vi "ACT_CLOSE.vi"(7 "StateValveModbus":T1=enum."CLOSING", 8 "error in (no error)":errorcluster, 11 "NeedleValve in":refnum<class "NeedleValve.lvclass">) -> (0 "error out":errorcluster, 3 "NeedleValve out":refnum<class "NeedleValve.lvclass">)   [LabVIEW 2019, in "NeedleValve.lvclass"]
uses:
  NeedleValve.lvclass
  TypeDef/Needle Valve State.ctl
  NeedleValve.lvclass/NeedleValve.ctl
  modbus engine custom/MB_ENGINE_class/cmd enum.ctl
  ef2003b6-d044-46f0-abe2-5d2387dde1d8.vi
  432cf372-d557-43cf-ab82-687c716dd17b.vi
  9ce69719-d540-4c82-92ba-c0e5243c761a.vi
  78836dd0-8225-4459-8d70-d600215e9411.vi
  modbus engine custom/MB_ENGINE_class/MB_ENGINE.lvclass
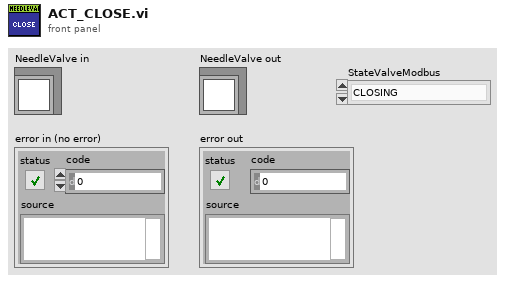
[diagram p1: front panel]
types:
  T1 = typedef "Needle Valve State.ctl" = enum16{"STOPED", "CLOSED", "OPENED", "OPENING", "CLOSING", "FULL_CLOSE"}
  T2 = typedef "MB_ENGINE.lvclass/cmd enum.ctl" = u16
  T3 = typedef "MB_ENGINE.lvclass/Settings.ctl" = cluster{"ACC Steps Per Sec^2":u16, "DEC Steps Per Sec^2":u16, "Min Velosity Step Per Sec":u16, "Max Velosity Step Per Sec":u16, "MicroStep":u16}
  T4 = typedef "Needle Valve Data.ctl" = cluster{"Engine State":T5, "StateValveModbus":T1, "Alarms":T6, "RAW":i32, "Angele":dbl, "Step":i32, "Encoder":i32, "Kinematic":T3, "Limits":T7, "EncoderMax":i32, "Counter Max Dont Update":i32, "EncoderMin":i32, "Counter Min Dont Update":i32, "Prepere Counter":i32, "STEP INIT":i32, "offset - Angel":dbl}
  T5 = typedef "MB_ENGINE.lvclass/Engine State.ctl" = u16
  T6 = typedef "MB_ENGINE.lvclass/Engine Alarms.ctl" = cluster{"OL":bool, "TF":bool, "STL":bool, "OCP":bool, "CPUV":bool, "UVLO":bool, "SPI_ERROR":bool, "Fault":bool, "OL 2":bool, "TF 2":bool, "STL 2":bool, "OCP 2":bool, "CPUV 2":bool, "UVLO 2":bool, "reserved":bool, "InitDone":bool}
  T7 = typedef "MB_ENGINE.lvclass/Limits Status.ctl" = cluster{"Fault 2 Switch":bool, "Fault 1 Switch":bool, "Center(Home)":bool, "Lower Limit":bool, "Upper Limit":bool}
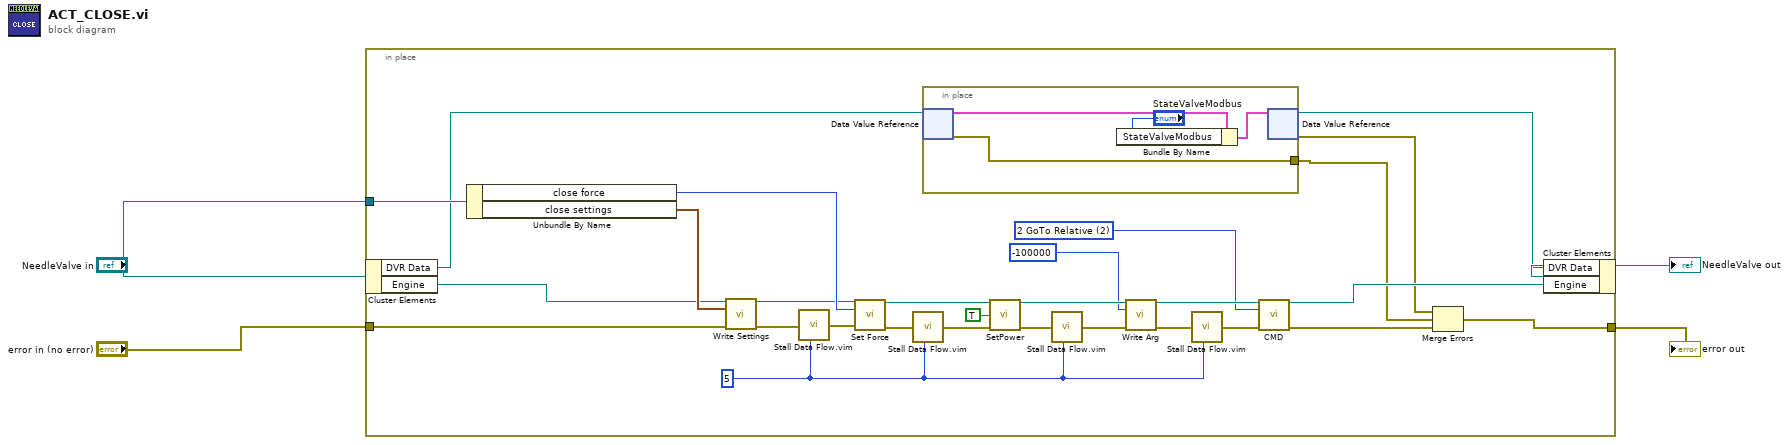
[diagram p0: block diagram]
diagram:
  n1 = in-place {
    in-place-border: "NeedleValve in" -> [w29]
    in-place-border: "error in (no error)" -> [w28]
    in-place-border: [w7] -> w3
    w19 = T2 2 items=["0 Idle"=0, "1 GoTo Absolute Position"=1, "2 GoTo Relative"=2, "10 GoTo Home Position"=10, "11 Set Home Position"=11, "12 Set FindHome Mode"=12, "13 Reset FindHome Mode"=13, "14 Get FindHome State"=14, "20 Hard Stop"=20, "21 HiZ Stop"=21, "22 Soft Stop"=22, "30 Clear Fault"=30, "40 Encoder Set Home"=40, "70 Driver Init"=70] ("cmd to write")
    w10 = u32 5 ("milliseconds to wait")
    n2 = in-place-cluster #1("NeedleValve in") -> ("DVR Data"=w9:refnum<data-value>, "Engine"=w27:refnum<class "MB_ENGINE.lvclass">)
    n3 = Unbundle By Name(w29) -> ("close force"=w31:u16, "close settings"=w30:T3)
    n4 = call "Write Settings.vi"("class data in"=w27, "cluster"=w30, "error in (no error)"=w28) -> ("class data out"=w26:refnum<class "MB_ENGINE.lvclass">, "error out"=w12:errorcluster)  [unwired: 11 in]
    n5 = call "Stall Data Flow.vim"("value in"=w12, "milliseconds to wait"=w10) -> ("value out"=w11:errorcluster)  [unwired: 1 out]
    n6 = call "Set Force.vi"("class data in"=w26, "percent"=w31, "error in (no error)"=w11) -> ("class data out"=w25:refnum<class "MB_ENGINE.lvclass">, "error out"=w24:errorcluster)  [unwired: 11 in]
    n7 = call "Stall Data Flow.vim"("value in"=w24, "milliseconds to wait"=w10) -> ("value out"=w23:errorcluster)  [unwired: 1 out]
    n8 = in-place {
      in-place-border: [w33] -> w5
      n9 = in-place-dvr #2(w9) -> (w36:T4, w33:errorcluster)
      n10 = Bundle By Name(cluster=w36, "StateValveModbus"="StateValveModbus") -> (w35:T4)
      n11 = in-place-dvr #2(w35) -> (w8:refnum<data-value>, w6:errorcluster)
    }
    n12 = call "SetPower.vi"("class data in"=w25, "On"=TRUE, "error in (no error)"=w23) -> ("class data out"=w16:refnum<class "MB_ENGINE.lvclass">, "error out"=w18:errorcluster)  [unwired: 11 in]
    n13 = call "Stall Data Flow.vim"("value in"=w18, "milliseconds to wait"=w10) -> ("value out"=w17:errorcluster)  [unwired: 1 out]
    n14 = call "Write Arg.vi"("class data in"=w16, "ARG U32"=-100000, "error in (no error)"=w17) -> ("class data out"=w20:refnum<class "MB_ENGINE.lvclass">, "error out"=w21:errorcluster)  [unwired: 11 in]
    n15 = call "Stall Data Flow.vim"("value in"=w21, "milliseconds to wait"=w10) -> ("value out"=w22:errorcluster)  [unwired: 1 out]
    n16 = call "CMD.vi"("class data in"=w20, "cmd to write"=w19, "error in (no error)"=w22) -> ("class data out"=w15:refnum<class "MB_ENGINE.lvclass">, "error out"=w14:errorcluster)  [unwired: 11 in]
    n17 = Merge Errors(w6, w5, w14) -> (w7:errorcluster)
    n18 = in-place-cluster #1("DVR Data"=w8, "Engine"=w15) -> (→"NeedleValve out":refnum<class "NeedleValve.lvclass">)
  }
  "error out" <- w3
